vi "Flush.vi"(8 "error in (no error)":errorcluster, 11 "Priority Message Queue in":refnum<class "Priority Message Queue.lvclass">) -> (0 "error out":errorcluster, 2 "Flushed Elements":refnum<class "Message.lvclass">[](array[class]), 3 "Priority Message Queue out":refnum<class "Priority Message Queue.lvclass">)   [LabVIEW 2020, in "Artifex.lvlib" / "Priority Message Queue.lvclass"]
uses:
  Priority Message Queue.lvclass
  Message/Message.lvclass
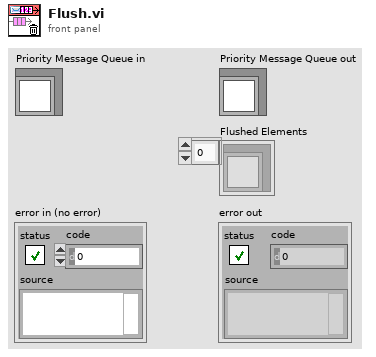
[diagram p1: front panel]
types:
  T1 = typedef "Artifex.lvlib/Priority Message Queue.lvclass/Ref Data.ctl" = cluster{"# Waiting":u32, "Buffers":refnum<queue>[], "Wait Msg":refnum<queue>, "Wait Prior":refnum<queue>}
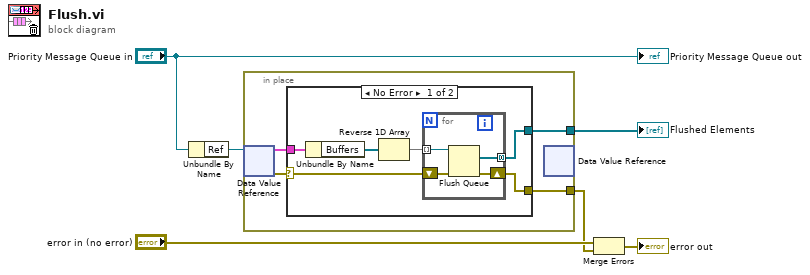
[diagram p0: block diagram]
diagram:
  n1 = Unbundle By Name("Priority Message Queue in") -> ("Ref"=w4:refnum<data-value>)
  n2 = in-place {
    in-place-border: [w8] -> w2
    in-place-border: [w7] -> w1
    n3 = in-place-dvr #1(w4) -> (w9:T1, w10:errorcluster)
    n4 = case shown="No Error" w10 {
      selector: w10 -> [w13 w21]
      tunnel: w9 -> [w16 _]
      tunnel: [w12 w21] -> w8
      tunnel: [w11 _] -> w7
      frame No Error {
        n5 = Unbundle By Name(w16) -> ("Buffers"=w15:refnum<queue>[])
        n6 = Reverse 1D Array(array=w15) -> (reversed array=w14:refnum<queue>[])
        n7 = for {
          tunnel: w14 -> [w20] mode=indexing
          tunnel: [w19] -> w11 mode=concatenating
          shift-right: [w18] -> w12
          shift-left: w13 -> [w17]
          n8 = Flush Queue(queue=w20, error in (no error)=w17) -> (remaining elements=w19:refnum<class "Message.lvclass">[], error out=w18:errorcluster)  [unwired: 1 out]
        }
      }
      frame Error {
      }
    }
    n9 = in-place-dvr #1() -> ()  [unwired: 1 in, 2 out]
  }
  "Flushed Elements" <- w1
  n10 = Merge Errors("error in (no error)", w2) -> (→"error out":errorcluster)
  "Priority Message Queue out" <- "Priority Message Queue in"
